vi "Set Configuration.vi"(8 "error in":errorcluster, 10 "Configuration":T1, 11 "Configuration in":refnum<class "Configuration.lvclass">) -> (0 "error out":errorcluster, 3 "Configuration out":refnum<class "Configuration.lvclass">)   [LabVIEW 2020, in "cycling structure demo UI.lvlib" / "Configuration.lvclass"]
doc: "____\nPeloton Config 2.0.0.6\nCopyright (c) 2024, Peloton"
uses:
  Configuration.lvclass
  Configuration--cluster.ctl
  Configuration.lvclass/Configuration.ctl
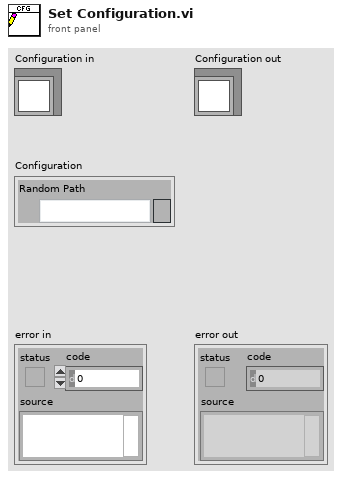
[diagram p1: front panel]
types:
  T1 = typedef "cycling structure demo UI.lvlib/Configuration.lvclass/Configuration--cluster.ctl" = cluster{"Random Path":path}
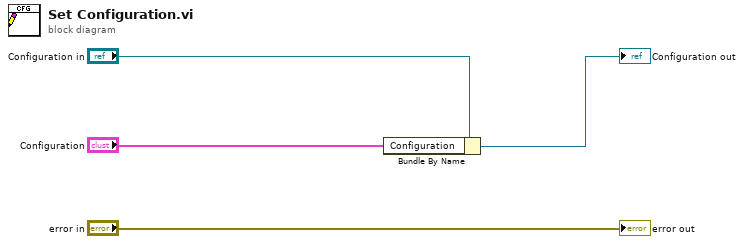
[diagram p0: block diagram]
diagram:
  n1 = Bundle By Name(cluster="Configuration in", "Configuration"="Configuration") -> (→"Configuration out":refnum<class "Configuration.lvclass">)
  "error out" <- "error in"
